vi "File Size.vi"(4 "文件大小（字节）":i64) -> (1 "文件大小（可读）":string)   [LabVIEW 2020]
doc: "名称 符号 二进制计量 十进制计量 字节数 等于\nKiloByte KB 2^10 10^3 1,024 1,024 B\nMegaByte MB 2^20 10^6 1,048,576 1,024 KB\nGigaByte GB 2^30 10^9 1,073,741,824 1,024 MB\nTeraByte TB 2^40 10^12 1,099,511,627,776 1,024 GB\nPetaByte PB 2^50 10^15 1,125,899,906,842,624 1,024 TB\nExaByte EB 2^60 10^18 1,152,921,504,606,846,976 1,024 PB"
panel:
  # "名称      符号 二进制计量  十进制计量   字节数                     等于\nKiloByte  KB   2^10       10^3        1,024                      1,024 B\nMegaByte  MB   2^20       10^6        1,048,576                  1,024 KB\nGigaByte  GB   2^30       10^9        1,073,741,824              1,024 MB\nTeraByte  TB   2^40       10^12       1,099,511,627,776          1,024 GB\nPetaByte  PB   2^50       10^15       1,125,899,906,842,624      1,024 TB\nExaByte   EB   2^60       10^18       1,152,921,504,606,846,976  1,024 PB"
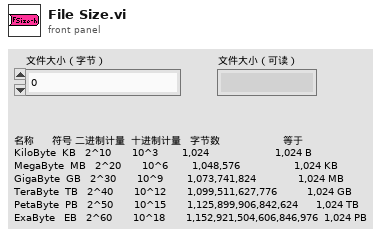
[diagram p1: front panel]
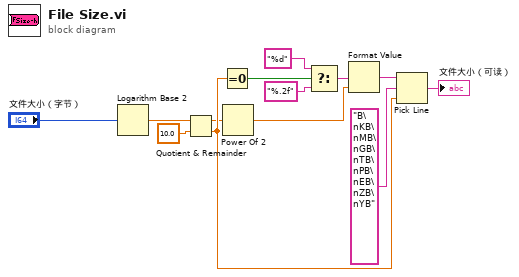
[diagram p0: block diagram]
diagram:
  n1 = Logarithm Base 2(1:"文件大小（字节）") -> (0:w13:dbl)
  n2 = Quotient & Remainder(x=w13, y=10.0) -> (x-y*floor(x/y)=w2:dbl, floor(x/y)=w11:dbl)
  n3 = Equal To 0?(x=w11) -> (x = 0?=w9:bool)
  n4 = Power Of 2(x=w2) -> (2^x=w1:dbl)
  n5 = Select(t="%d" ("格式字符串"), s=w9, f="%.2f") -> (s? t:f=w6:string)
  n6 = Format Value(format string=w6, value (0)=w1) -> (output string=w5:string)  [unwired: 1 in]
  n7 = Pick Line(string ("")=w5, multi-line string="B\nKB\nMB\nGB\nTB\nPB\nEB\nZB\nYB" ("电子表格字符串"), line index=w11) -> (output string=→"文件大小（可读）":string)
